vi "Set Colors.vi"(8 "error in":errorcluster, 9 "Color 2":T1, 10 "Color 1":T1, 11 "Cell View Back Color Alternate in":refnum<class "Cell View Back Color Alternate.lvclass">) -> (0 "error out":errorcluster, 3 "Cell View Back Color Alternate out":refnum<class "Cell View Back Color Alternate.lvclass">)   [LabVIEW 2024, in "PDO Grid.lvlib" / "Cell View Back Color Alternate.lvclass"]
uses:
  Cell View Back Color Alternate.lvclass
  Cell View Back Color Alternate.lvclass/Cell View Back Color Alternate.ctl
  Sourcegrid-LabVIEW/source/Color/Color.lvclass
  Sourcegrid-LabVIEW/source/System.Drawing.Color.ctl
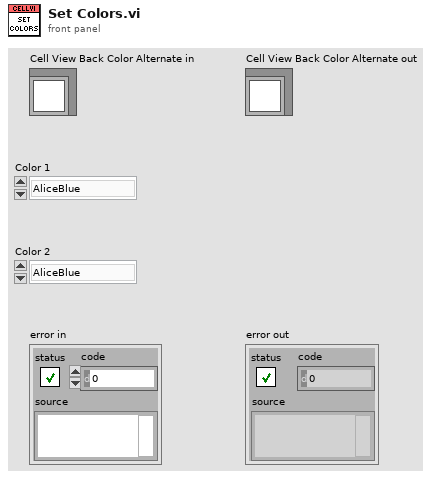
[diagram p1: front panel]
types:
  T1 = typedef "System.Drawing.Color.ctl" = enum16{"AliceBlue", "AntiqueWhite", "Aqua", "Aquamarine", "Azure", "Beige", "Bisque", "Black", "BlanchedAlmond", "Blue", "BlueViolet", "Brown", "BurlyWood", "CadetBlue", "Chartreuse", "Chocolate", "Coral", "CornflowerBlue", "Cornsilk", "Crimson", "Cyan", "DarkBlue", "DarkCyan", "DarkGoldenrod", "DarkGray", "DarkGreen", "DarkKhaki", "DarkMagenta", "DarkOliveGreen", "DarkOrange", "DarkOrchid", "DarkRed", "DarkSalmon", "DarkSeaGreen", "DarkSlateBlue", "DarkSlateGray", "DarkTurquoise", "DarkViolet", "DeepPink", "DeepSkyBlue", "DimGray", "DodgerBlue", "Firebrick", "FloralWhite", "ForestGreen", "Fuchsia", "Gainsboro", "GhostWhite", "Gold", "Goldenrod", "Gray", "Green", "GreenYellow", "Honeydew", "HotPink", "IndianRed", "Indigo", "Ivory", "Khaki", "Lavender", "LavenderBlush", "LawnGreen", "LemonChiffon", "LightBlue", "LightCoral", "LightCyan", "LightGoldenrodYellow", "LightGray", "LightGreen", "LightPink", "LightSalmon", "LightSeaGreen", "LightSkyBlue", "LightSlateGray", "LightSteelBlue", "LightYellow", "Lime", "LimeGreen", "Linen", "Magenta", "Maroon", "MediumAquamarine", "MediumBlue", "MediumOrchid", "MediumPurple", "MediumSeaGreen", "MediumSlateBlue", "MediumSpringGreen", "MediumTurquoise", "MediumVioletRed", "MidnightBlue", "MintCream", "MistyRose", "Moccasin", "NavajoWhite", "Navy", "OldLace", "Olive", "OliveDrab", "Orange", "OrangeRed", "Orchid", "PaleGoldenrod", "PaleGreen", "PaleTurquoise", "PaleVioletRed", "PapayaWhip", "PeachPuff", "Peru", "Pink", "Plum", "PowderBlue", "Purple", "Red", "RosyBrown", "RoyalBlue", "SaddleBrown", "Salmon", "SandyBrown", "SeaGreen", "SeaShell", "Sienna", "Silver", "SkyBlue", "SlateBlue", "SlateGray", "Snow", "SpringGreen", "SteelBlue", "Tan", "Teal", "Thistle", "Tomato", "Transparent", "Turquoise", "Violet", "Wheat", "White", "WhiteSmoke", "Yellow"}
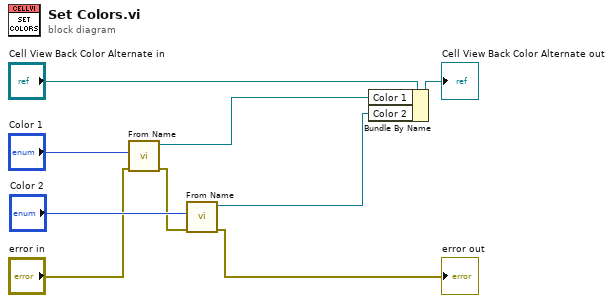
[diagram p0: block diagram]
diagram:
  n1 = call "From Name.vi"("error in"="error in", "Color"="Color 1") -> ("error out"=w5:errorcluster, "Color out"=w3:refnum<class "Color.lvclass">)  [unwired: 8 in]
  n2 = call "From Name.vi"("error in"=w5, "Color"="Color 2") -> ("error out"=→"error out":errorcluster, "Color out"=w2:refnum<class "Color.lvclass">)  [unwired: 8 in]
  n3 = Bundle By Name(cluster="Cell View Back Color Alternate in", "Color 1"=w3, "Color 2"=w2) -> (→"Cell View Back Color Alternate out":refnum<class "Cell View Back Color Alternate.lvclass">)
